vi "get_or_set_modifier_values.vi"(5 "modifier index":i32, 6 "clamp output values?":bool[](array[boolean]), 7 "action":T1, 8 "error in (no error)":errorcluster, 10 "modifier values in":dbl[](array[numeric]), 11 "GenericTrajectory in":refnum<class "TrajectoryDL091126GenericVoxel.lvclass">) -> (0 "error out":errorcluster, 2 "modifier values out":dbl[](array[numeric]), 3 "GenericTrajectory out":refnum<class "TrajectoryDL091126GenericVoxel.lvclass">)   [LabVIEW 2010, in "TrajectoryDL091126GenericVoxel.lvclass"]
uses:
  TrajectoryDL091126GenericVoxel.lvclass
  common/enumerations/functional_global_action_enum.ctl
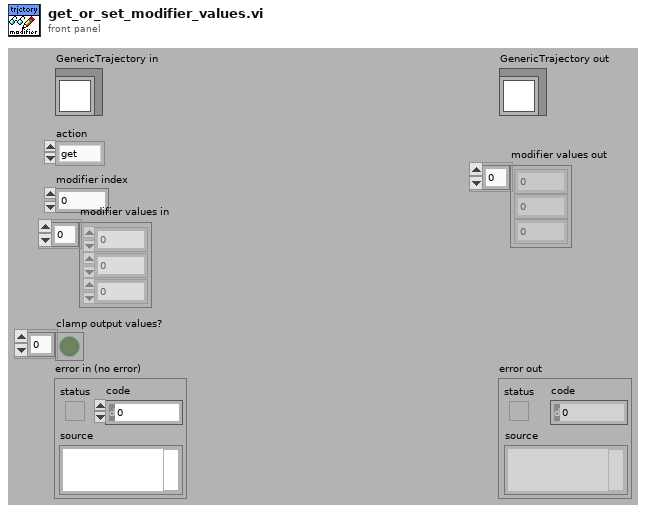
[diagram p1: front panel]
types:
  T1 = typedef "functional_global_action_enum.ctl" = enum16{"get", "set", "reset"}
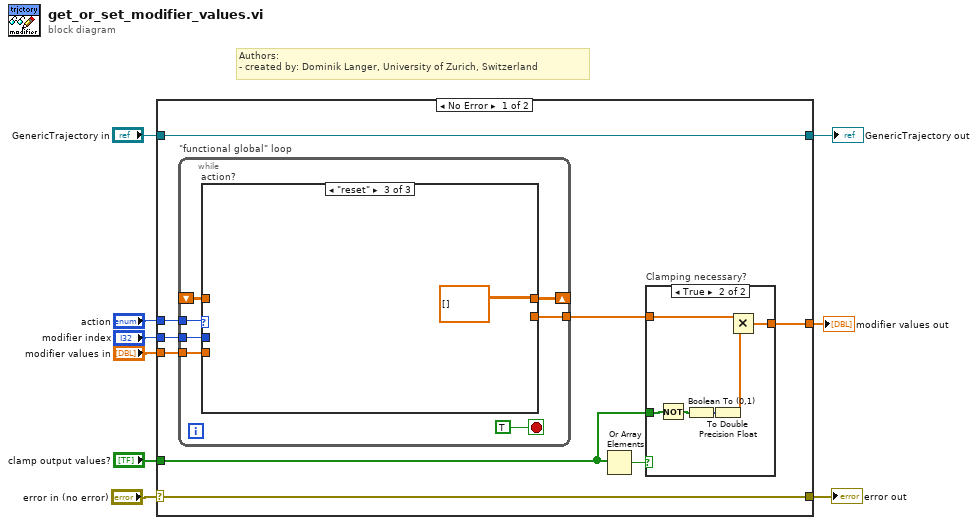
[diagram p0: block diagram]
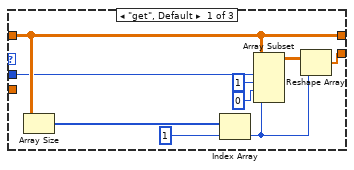
[diagram p3: hidden frame]
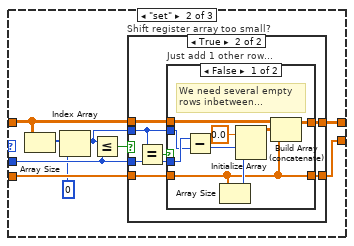
[diagram p4: hidden frame]
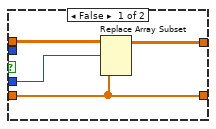
[diagram p5: hidden frame]
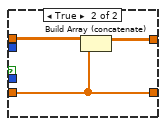
[diagram p6: hidden frame]
diagram:
  # "Authors: \n- created by: Dominik Langer, University of Zurich, Switzerland"
  n1 = case shown="No Error" "error in (no error)" {
    selector: "error in (no error)" -> [w17 w76]
    tunnel: [w17 w76] -> w8
    tunnel: [w18 w75] -> w6
    tunnel: "GenericTrajectory in" -> [w18 w75]
    tunnel: "modifier index" -> [w15 _]
    tunnel: "action" -> [w16 _]
    tunnel: "modifier values in" -> [w14 _]
    tunnel: [w11 _] -> w2
    tunnel: "clamp output values?" -> [w10 _]
    frame No Error {
      n2 = while "\"functional global\" loop" {
        tunnel: w15 -> [w32]
        tunnel: [w31] -> w12
        tunnel: w16 -> [w28]
        shift-right: [w29] -> _
        shift-left: _ -> [w30]
        tunnel: w14 -> [w27]
        stop <- TRUE stop-if-true
        n3 = case "action?" shown="\"reset\"" w28 {
          tunnel: w32 -> [w35 w46 _]
          tunnel: [w41 w42 _] -> w31
          tunnel: w30 -> [w38 w48 _]
          tunnel: [w38 w50 dbl[][] [] ("modifier values in")] -> w29
          tunnel: w27 -> [_ w49 _]
          frame "get", Default {
            n4 = Array Size(array=w38) -> (size(s)=w36:i32[])
            n5 = Index Array(array=w36, index=1) -> (element=w34:i32)
            n6 = Array Subset(array=w38, index (row)=w35, length (row)=1 ("length"), index (col)=0 ("index"), length (col)=w34) -> (w40:dbl[][])
            n7 = Reshape Array(w40, w34) -> (w41:dbl[])
          }
          frame "set" {
            n8 = Array Size(array=w48) -> (size(s)=w45:i32[])
            n9 = Index Array(array=w45, index=0) -> (element=w43:i32)
            n10 = Less Or Equal?(x=w43, y=w46) -> (x <= y?=w47:bool)
            n11 = case "Shift register array too small?" shown="True" w47 {
              tunnel: w48 -> [w54 w60]
              tunnel: [w53 w58] -> w50
              tunnel: w46 -> [w52 w57]
              tunnel: w49 -> [w51 w59]
              tunnel: w43 -> [_ w56]
              tunnel: [w51 w55] -> w42
              frame False {
                n12 = Replace Array Subset(array=w54, new element=w51, index (row)=w52) -> (w53:dbl[][])  [unwired: 1 in]
              }
              frame True {
                n13 = Equal?(x=w56, y=w57) -> (x = y?=w61:bool)
                n14 = case "Just add 1 other row..." shown="False" w61 {
                  tunnel: w60 -> [w70 w73]
                  tunnel: w59 -> [w62 w72]
                  tunnel: [w69 w71] -> w58
                  tunnel: w57 -> [w65 _]
                  tunnel: w56 -> [w64 _]
                  tunnel: [w62 w72] -> w55
                  frame False {
                    # "We need several empty rows inbetween..."
                    n15 = Subtract(x=w65, y=w64) -> (x-y=w63:i32)
                    n16 = Array Size(array=w62) -> (size(s)=w66:i32)
                    n17 = Initialize Array(0.0 ("element"), w63, w66) -> (w68:dbl[][])
                    n18 = Build Array (concatenate)(w70, w68, w62) -> (w69:dbl[][])
                  }
                  frame True {
                    n19 = Build Array (concatenate)(w73, w72) -> (w71:dbl[][])
                  }
                }
              }
            }
          }
          frame "reset" {
          }
        }
      }
      n20 = Or Array Elements(Boolean array=w10) -> (logical OR=w13:bool)
      n21 = case "Clamping necessary?" shown="True" w13 {
        tunnel: [w19 w25] -> w11
        tunnel: w12 -> [w19 w24]
        tunnel: w10 -> [_ w21]
        frame False {
        }
        frame True {
          n22 = Not(x=w21) -> (.not. x?=w20:bool[])
          n23 = Boolean To (0,1)(Boolean=w20) -> (0, 1=w23:i16[])
          n24 = To Double Precision Float(number=w23) -> (double precision float=w22:dbl[])
          n25 = Multiply(x=w24, y=w22) -> (x*y=w25:dbl[])
        }
      }
    }
    frame Error {
    }
  }
  "error out" <- w8
  "GenericTrajectory out" <- w6
  "modifier values out" <- w2
